vi "MISC Find_All_Files_And_Folders.vi"(0 "High Level Directory":path, 5 "pattern (*.*)":string="*.*", 11 "error in (no error)":errorcluster) -> (4 "All File Paths":path[](array[path]), 6 "All Directory Paths":path[](array[path]), 8 "number of files":i32, 10 "number of directories":i32, 15 "error out":errorcluster)   [LabVIEW 2011]
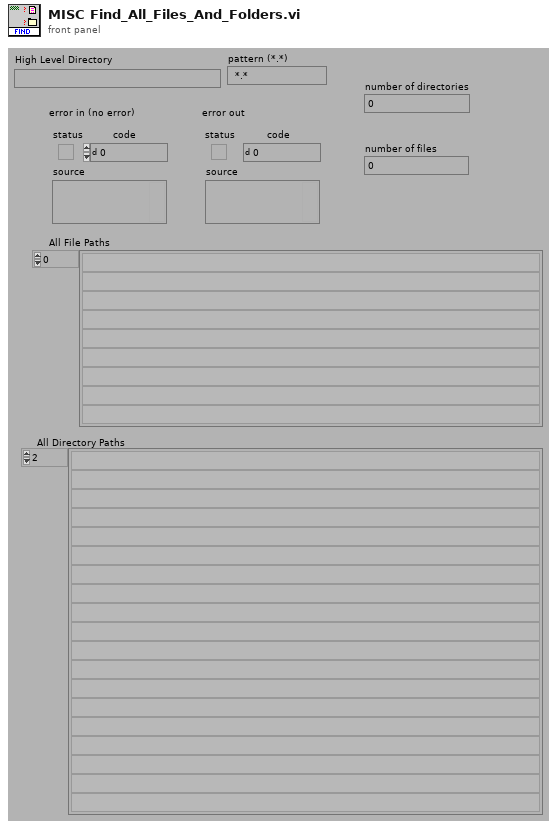
[diagram p1: front panel]
types:
  T1 = enum32{"existing file", "new file", "new or existing file", "existing dir", "new dir", "new or existing dir", "existing file (use LLBs)", "new file (use LLBs)", "new or existing file (use LLBs)", "new or existing file or directory (use LLBs)"}
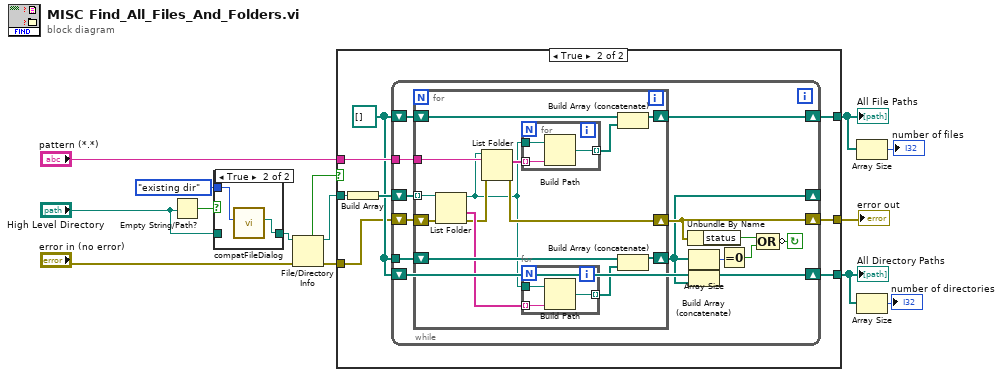
[diagram p0: block diagram]
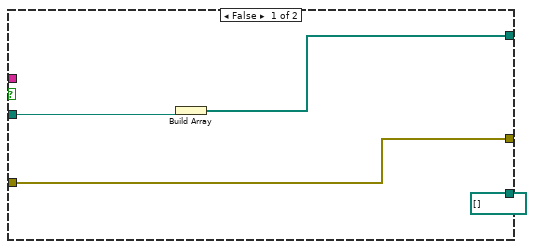
[diagram p2: hidden frame]
diagram:
  n1 = Empty String/Path?(string/path="High Level Directory") -> (empty?=w12:bool)
  n2 = case shown="True" w12 {
    tunnel: [w15 w17] -> w4
    tunnel: "High Level Directory" -> [w15 _]
    tunnel: T1."existing dir" ("select mode (2)") -> [_ w16]
    frame False {
    }
    frame True {
      n3 = call <vilib>:"compatFileDialog.vi"("select mode (2)"=w16) -> ("path"=w17:path)  [unwired: 6 in, 4 out]
    }
  }
  n4 = File/Directory Info(path=w4, error in="error in (no error)") -> (path out=w3:path, directory=w2:bool, error out=w1:errorcluster)  [unwired: 4 out]
  n5 = case shown="True" w2 {
    tunnel: [w18 w28] -> w14
    tunnel: [w19 w27] -> w13
    tunnel: "pattern (*.*)" -> [_ w26]
    tunnel: [path[] [] w25] -> w8
    tunnel: w3 -> [w20 w24]
    tunnel: w1 -> [w18 w22]
    frame False {
      n6 = Build Array(w20) -> (w19:path[])
    }
    frame True {
      w23 = path[] []
      n7 = Build Array(w24) -> (w29:path[])
      n8 = while {
        shift-left: w23 -> [w31]
        shift-right: [w32] -> w25
        tunnel: w26 -> [w34]
        shift-left: w22 -> [w39]
        shift-right: [w38] -> w28
        shift-left: w23 -> [w36]
        shift-right: [w35] -> w27
        shift-left: w29 -> [w43]
        shift-right: [w30] -> _
        tunnel: w23 -> [w33]
        stop <- w40 continue-if-true
        n9 = for {
          tunnel: w43 -> [w54] mode=indexing
          shift-right: [w46] -> w38
          shift-left: w39 -> [w57]
          shift-right: [w56] -> w30
          shift-left: w33 -> [w55]
          shift-right: [w50] -> w35
          shift-left: w36 -> [w51]
          tunnel: w34 -> [w49]
          n10 = List Folder(path=w54, error in=w57) -> (path out=w44:path, folder names=w53:string[], error out=w47:errorcluster)  [unwired: 3 out]
          n11 = List Folder(path=w44, pattern=w49, error in=w47) -> (filenames=w48:string[], error out=w46:errorcluster)  [unwired: 3 out]
          n12 = for {
            tunnel: w44 -> [w60]
            tunnel: [w59] -> w52 mode=indexing
            tunnel: w48 -> [w58] mode=indexing
            n13 = Build Path(base path=w60, name or relative path=w58) -> (appended path=w59:path)
          }
          n14 = for {
            tunnel: w44 -> [w63]
            tunnel: w53 -> [w62] mode=indexing
            tunnel: [w61] -> w45 mode=indexing
            n15 = Build Path(base path=w63, name or relative path=w62) -> (appended path=w61:path)
          }
          n16 = Build Array (concatenate)(w51, w52) -> (w50:path[])
          n17 = Build Array (concatenate)(w55, w45) -> (w56:path[])
        }
        n18 = Unbundle By Name(w38) -> ("status"=w42:bool)
        n19 = Array Size(array=w30) -> (size(s)=w37:i32)
        n20 = Build Array (concatenate)(w31, w30) -> (w32:path[])
        n21 = Equal To 0?(x=w37) -> (x = 0?=w41:bool)
        n22 = Compound Arithmetic op=OR(w42, w41) -> (invert w40:bool)
      }
    }
  }
  "error out" <- w14
  "All File Paths" <- w13
  "All Directory Paths" <- w8
  n23 = Array Size(array=w13) -> (size(s)=→"number of files":i32)
  n24 = Array Size(array=w8) -> (size(s)=→"number of directories":i32)
